vi "GUI Open Synchronization Objects.vi"(8 "error in (no error)":errorcluster) -> (0 "error out":errorcluster, 3 "FOFB GUI":T1)   [LabVIEW 2011, in "User Interface VIs.lvlib"]
uses:
  User Interface VIs.lvlib
  Types Definitions/Type FOFB GUI.ctl
  Types Definitions/Type Configuration Data (GUI to Controller).ctl
  Types Definitions/Type Monitoring Data.ctl
  Types Definitions/Type Diagnostics Data.ctl
  Types Definitions/Type CPU Loads Array.ctl
  Types Definitions/Type CPU Loads.ctl
  Types Definitions/Type Diagnostics Sample.ctl
  Types Definitions/Type Monitoring Sample.ctl
  Type Definitions.lvlib
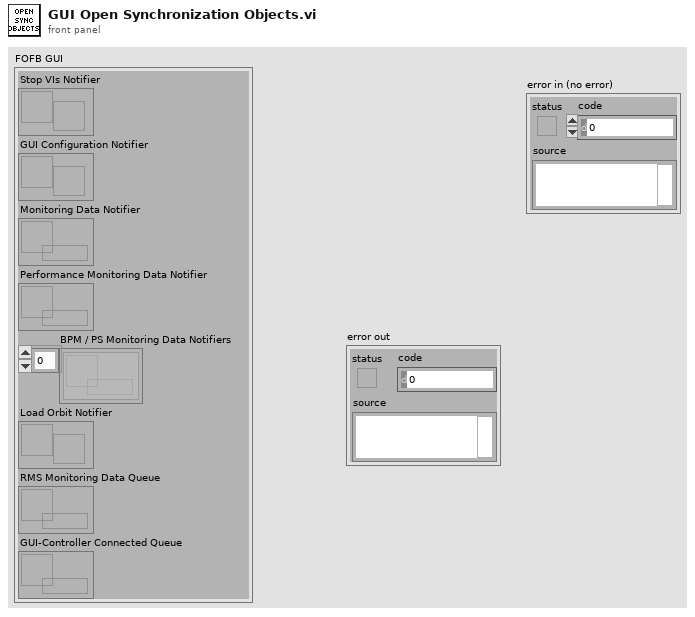
[diagram p1: front panel]
types:
  T1 = typedef "Type Definitions.lvlib/Type FOFB GUI.ctl" = cluster{"Stop VIs Notifier":refnum<notifier>, "GUI Configuration Notifier":refnum<notifier>, "Monitoring Data Notifier":refnum<queue>, "Performance Monitoring Data Notifier":refnum<queue>, "BPM / PS Monitoring Data Notifiers":refnum<queue>[], "Load Orbit Notifier":refnum<notifier>, "RMS Monitoring Data Queue":refnum<queue>, "GUI-Controller Connected Queue":refnum<queue>}
  T2 = typedef "Type Definitions.lvlib/Type Configuration Data (GUI to Controller).ctl" = cluster{"Operation Mode":enum16{"Idle Mode", "Error Mode", "Manual Mode", "FOFB Mode", "RMM Mode"}[], "Update Controller Soft Configuration":bool[], "Trigger RT Execution Trace":string[]}
  T3 = typedef "Type Definitions.lvlib/Type Diagnostics Sample.ctl" = cluster{"Timestamp":timestamp, "Diagnostics Data":T4}
  T4 = typedef "Type Definitions.lvlib/Type Diagnostics Data.ctl" = cluster{"Time-Critical Loop Missed Iterations":u32, "Time-Critical Loop Execution Time (usec)":u32, "FA Buffer Usage":u32, "Available Memory (bytes)":u32, "CPU Loads Array":T5}
  T5 = typedef "Type Definitions.lvlib/Type CPU Loads Array.ctl" = T6[]
  T6 = typedef "Type Definitions.lvlib/Type CPU Loads.ctl" = cluster{"Total (%)":dbl, "Time Critical (%)":dbl, "Timed Structures (%)":dbl, "High (%)":dbl, "Above Normal (%)":dbl, "Normal (%)":dbl, "Background (%)":dbl, "Idle (%)":dbl, "ISR (%)":dbl}
  T7 = typedef "Type Definitions.lvlib/Type Monitoring Sample.ctl" = cluster{"Timestamp":timestamp, "Sample":dbl[]}
  T8 = typedef "Type Definitions.lvlib/Type Monitoring Data.ctl" = cluster{"Timestamp":timestamp, "BPM Readings":dbl[], "PS Readings":dbl[], "PS FOFB Setpoints":dbl[], "PS Status per Rack":u8[], "PS ON-OFF per Rack":u8[], "Operation Mode":enum16{"Idle Mode", "Error Mode", "Manual Mode", "FOFB Mode", "RMM Mode"}, "Diagnostics Data":T4, "Controller Status Table":i32[]}
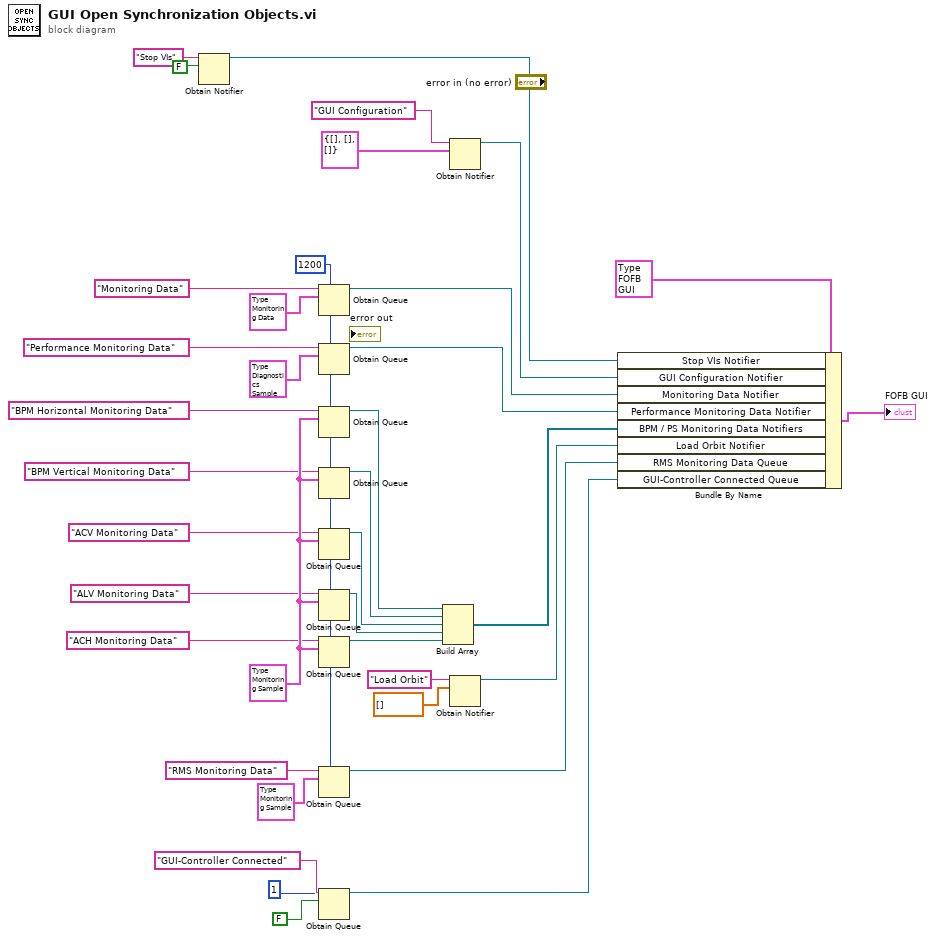
[diagram p0: block diagram]
diagram:
  w25 = T7 {"Timestamp"=timestamp(0 s since 1904-01-01), "Sample"=[]} ("Monitoring Sample")
  w1 = 1200 ("max queue size (-1, unlimited)")
  n1 = Obtain Notifier(name (unnamed)="Stop VIs", notification data type=FALSE) -> (notifier out=w29:refnum<notifier>)  [unwired: 2 in, 2 out]
  n2 = Obtain Queue(max queue size (-1, unlimited)=w1, name (unnamed)="Monitoring Data", element data type=T8 {"Timestamp"=timestamp(0 s since 1904-01-01), "BPM Readings"=[], "PS Readings"=[], "PS FOFB Setpoints"=[], "PS Status per Rack"=[], "PS ON-OFF per Rack"=[], "Operation Mode"=enum."Idle Mode", "Diagnostics Data"={"Time-Critical Loop Missed Iterations"=0, "Time-Critical Loop Execution Time (usec)"=0, "FA Buffer Usage"=0, "Available Memory (bytes)"=0, "CPU Loads Array"=[]}, "Controller Status Table"=[]} ("Slow Data")) -> (queue out=w31:refnum<queue>)  [unwired: 2 in, 2 out]
  n3 = Obtain Queue(max queue size (-1, unlimited)=w1, name (unnamed)="Performance Monitoring Data", element data type=T3 {"Timestamp"=timestamp(0 s since 1904-01-01), "Diagnostics Data"={"Time-Critical Loop Missed Iterations"=0, "Time-Critical Loop Execution Time (usec)"=0, "FA Buffer Usage"=0, "Available Memory (bytes)"=0, "CPU Loads Array"=[]}} ("Diagnostics  Sample")) -> (queue out=w32:refnum<queue>)  [unwired: 2 in, 2 out]
  n4 = Obtain Queue(max queue size (-1, unlimited)=w1, name (unnamed)="BPM Horizontal Monitoring Data", element data type=w25) -> (queue out=w18:refnum<queue>)  [unwired: 2 in, 2 out]
  n5 = Obtain Queue(max queue size (-1, unlimited)=w1, name (unnamed)="BPM Vertical Monitoring Data", element data type=w25) -> (queue out=w19:refnum<queue>)  [unwired: 2 in, 2 out]
  n6 = Obtain Queue(max queue size (-1, unlimited)=w1, name (unnamed)="ACV Monitoring Data", element data type=w25) -> (queue out=w20:refnum<queue>)  [unwired: 2 in, 2 out]
  n7 = Obtain Queue(max queue size (-1, unlimited)=w1, name (unnamed)="ALV Monitoring Data", element data type=w25) -> (queue out=w21:refnum<queue>)  [unwired: 2 in, 2 out]
  n8 = Obtain Queue(max queue size (-1, unlimited)=w1, name (unnamed)="ACH Monitoring Data", element data type=w25) -> (queue out=w24:refnum<queue>)  [unwired: 2 in, 2 out]
  n9 = Obtain Queue(max queue size (-1, unlimited)=w1, name (unnamed)="RMS Monitoring Data", element data type=T7 {"Timestamp"=timestamp(0 s since 1904-01-01), "Sample"=[]} ("Monitoring Sample")) -> (queue out=w37:refnum<queue>)  [unwired: 2 in, 2 out]
  n10 = Obtain Queue(max queue size (-1, unlimited)=1, name (unnamed)="GUI-Controller Connected", element data type=FALSE) -> (queue out=w4:refnum<queue>)  [unwired: 2 in, 2 out]
  n11 = Build Array(w18, w19, w20, w21, w24) -> (w33:refnum<queue>[])
  n12 = Obtain Notifier(name (unnamed)="GUI Configuration", notification data type=T2 {"Operation Mode"=[], "Update Controller Soft Configuration"=[], "Trigger RT Execution Trace"=[]} ("Configuration Data (GUI to Controller)")) -> (notifier out=w30:refnum<notifier>)  [unwired: 2 in, 2 out]
  n13 = Obtain Notifier(name (unnamed)="Load Orbit", notification data type=dbl[] [] ("initialized array")) -> (notifier out=w36:refnum<notifier>)  [unwired: 2 in, 2 out]
  n14 = Bundle By Name(cluster=T1 {"Stop VIs Notifier"=refnum, "GUI Configuration Notifier"=refnum, "Monitoring Data Notifier"=refnum, "Performance Monitoring Data Notifier"=refnum, "BPM / PS Monitoring Data Notifiers"=[], "Load Orbit Notifier"=refnum, "RMS Monitoring Data Queue"=refnum, "GUI-Controller Connected Queue"=refnum} ("FOFB GUI"), "Stop VIs Notifier"=w29, "GUI Configuration Notifier"=w30, "Monitoring Data Notifier"=w31, "Performance Monitoring Data Notifier"=w32, "BPM / PS Monitoring Data Notifiers"=w33, "Load Orbit Notifier"=w36, "RMS Monitoring Data Queue"=w37, "GUI-Controller Connected Queue"=w4) -> (→"FOFB GUI":T1)
